vi "LM79 Stabilization.vi"(8 "error in (no error)":errorcluster, 10 "Time Between\nMeasurements (s)":dbl, 11 "Data over time":dbl[](array[numeric])) -> (0 "error out":errorcluster, 1 "Stabilization Data Out":T1, 2 "Stabilized":bool)   [LabVIEW 2014, in "Timing and Stabilization.lvlib"]
uses:
  Timing and Stabilization.lvlib
  Stabilization.ctl
  avantesSpectrometer/Acquisition/Sphere Indicator.ctl
  <vilib>/Analysis/baseanly.llb/Mean (DBL).vi
  <vilib>/Analysis/NI_AALBase.lvlib
  avantesSpectrometer/AvaSpec.lvlib
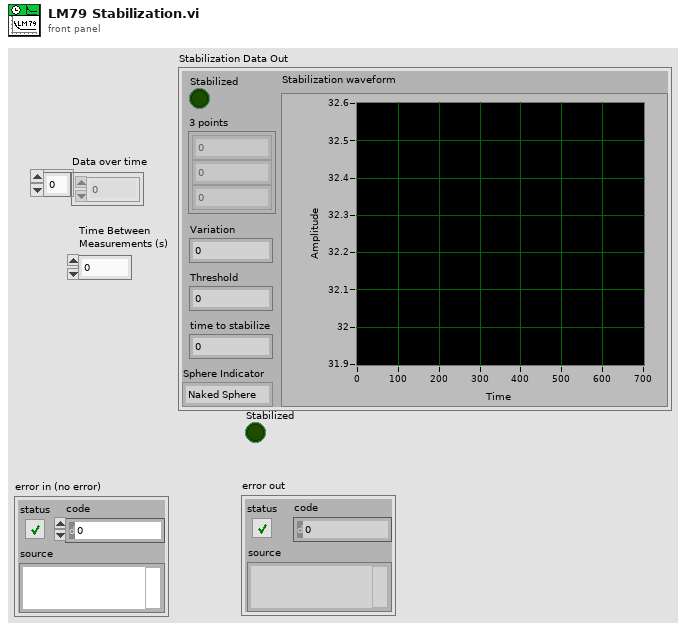
[diagram p1: front panel]
types:
  T1 = typedef "Timing and Stabilization.lvlib/Stabilization.ctl" = cluster{"Stabilization waveform":waveform(dbl), "Variation":dbl, "Stabilized":bool, "Threshold":dbl, "time to stabilize":dbl, "3 points":dbl[], "Sphere Indicator":T2}
  T2 = typedef "AvaSpec.lvlib/Sphere Indicator.ctl" = enum16{"Naked Sphere", "Insulated Sphere"}
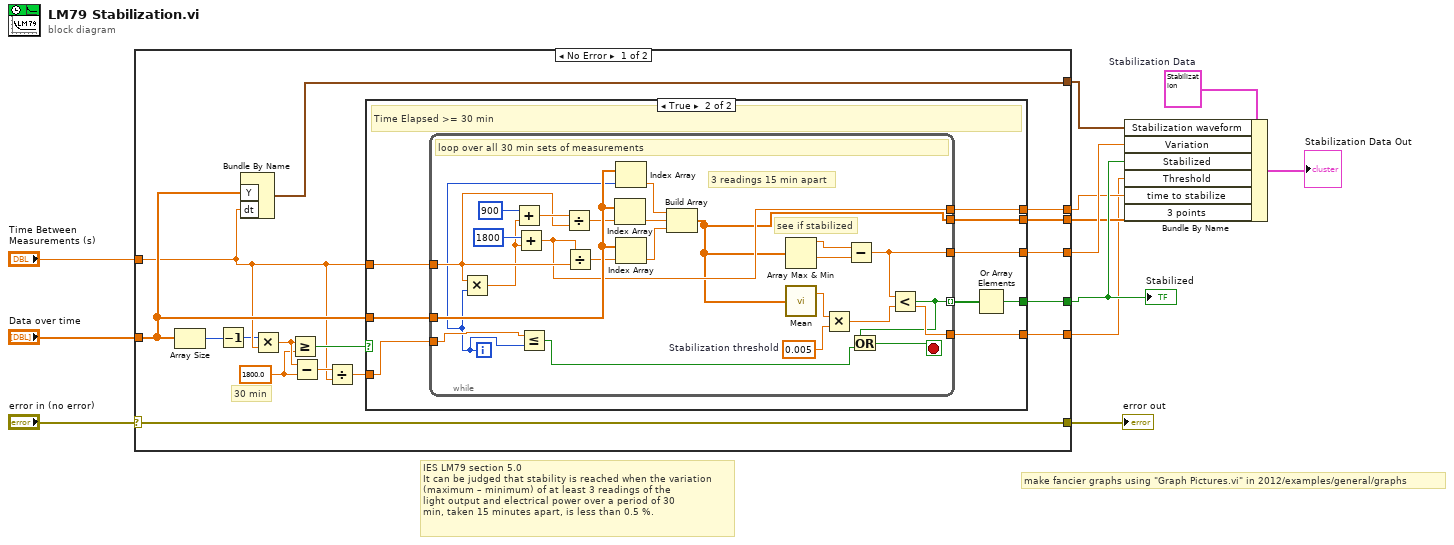
[diagram p0: block diagram]
diagram:
  w8 = T1 {"Stabilization waveform"={"t0"=timestamp(0 s since 1904-01-01), "dt"=1.0, "Y"=[]}, "Variation"=0.0, "Stabilized"=FALSE, "Threshold"=0.0, "time to stabilize"=0.0, "3 points"=[], "Sphere Indicator"=enum."Naked Sphere"}  # Stabilization Data
  # "make fancier graphs using \"Graph Pictures.vi\" in 2012/examples/general/graphs"
  # "IES LM79 section 5.0\nIt can be judged that stability is reached when the variation\n(maximum – minimum) of at least 3 readings of the\nlight output and electrical power over a period of 30\nmin, taken 15 minutes apart, is less than 0.5 %."
  n1 = case shown="No Error" "error in (no error)" {
    selector: "error in (no error)" -> [w28 w62]
    tunnel: [w28 w62] -> w11
    tunnel: "Data over time" -> [w24 _]
    tunnel: "Time Between\nMeasurements (s)" -> [w17 _]
    tunnel: [w26 _] -> w7
    tunnel: [w25 _] -> w5
    tunnel: [w19 _] -> w6
    tunnel: [w18 _] -> w2
    tunnel: [w16 _] -> w3
    tunnel: [w15 _] -> w4
    frame No Error {
      w22 = 1800.0 ("y")
      # "30 min"
      n2 = Array Size(array=w24) -> (size(s)=w14:i32)
      n3 = Decrement(x=w14) -> (x-1=w13:i32)
      n4 = Bundle By Name("Y"=w24, "dt"=w17) -> (w26:waveform(dbl))  [unwired: 1 in]
      n5 = Multiply(x=w13, y=w17) -> (x*y=w23:dbl)
      n6 = Greater Or Equal?(x=w23, y=w22) -> (x >= y?=w27:bool)
      n7 = Subtract(x=w23, y=w22) -> (x-y=w21:dbl)
      n8 = Divide(x=w21, y=w17) -> (x/y=w20:dbl)
      n9 = case shown="True" w27 {
        tunnel: [_ w34] -> w25
        tunnel: w24 -> [_ w37]
        tunnel: w20 -> [_ w31]
        tunnel: w17 -> [_ w36]
        tunnel: [_ w33] -> w19
        tunnel: [_ w32] -> w18
        tunnel: [_ w30] -> w16
        tunnel: [_ w29] -> w15
        frame False {
        }
        frame True {
          # "Time Elapsed >= 30 min"
          n10 = while {
            tunnel: [w41] -> w35 mode=indexing
            tunnel: w37 -> [w57]
            tunnel: w36 -> [w50]
            tunnel: [w47] -> w33
            tunnel: [w46] -> w32
            tunnel: w31 -> [w44]
            tunnel: [w39] -> w30
            tunnel: [w38] -> w29
            i -> [w43]
            stop <- w45 stop-if-true
            w58 = 0.005  # Stabilization threshold
            # "3 readings 15 min apart"
            # "see if stabilized"
            # "loop over all 30 min sets of measurements"
            n11 = Multiply(x=w50, y=w43) -> (x*y=w40:dbl)
            n12 = Add(x=900, y=w40) -> (x+y=w52:dbl)
            n13 = Add(x=1800, y=w40) -> (x+y=w39:dbl)
            n14 = Less Or Equal?(x=w44, y=w43) -> (x <= y?=w42:bool)
            n15 = Divide(x=w52, y=w50) -> (x/y=w48:dbl)
            n16 = Divide(x=w39, y=w50) -> (x/y=w49:dbl)
            n17 = Index Array(array=w57, index=w48) -> (element=w55:dbl)
            n18 = Index Array(array=w57, index=w43) -> (element=w56:dbl)
            n19 = Index Array(array=w57, index=w49) -> (element=w54:dbl)
            n20 = Build Array(w56, w55, w54) -> (w38:dbl[])
            n21 = Array Max & Min(array=w38) -> (max value=w61:dbl, min value=w60:dbl)  [unwired: 2 out]
            n22 = call-poly <vilib>:"Mean.vi"("X"=w38) -> ("mean"=w59:dbl)  [unwired: 1 out]
            n23 = Multiply(x=w59, y=w58) -> (x*y=w46:dbl)
            n24 = Subtract(x=w61, y=w60) -> (x-y=w47:dbl)
            n25 = Less?(x=w47, y=w46) -> (x < y?=w41:bool)
            n26 = Or(x=w41, y=w42) -> (x .or. y?=w45:bool)
          }
          n27 = Or Array Elements(Boolean array=w35) -> (logical OR=w34:bool)
        }
      }
    }
    frame Error {
    }
  }
  "error out" <- w11
  "Stabilized" <- w5
  n28 = Bundle By Name(cluster=w8, "Stabilization waveform"=w7, "Variation"=w6, "Stabilized"=w5, "Threshold"=w2, "time to stabilize"=w3, "3 points"=w4) -> (→"Stabilization Data Out":T1)
